vi "SECoP-filterStoredCommand_2.vi"(8 "error in (no error)":errorcluster, 9 "filter action":T1, 10 "filter accessibles":string[](array[string]), 11 "DLL path (in)":T2) -> (0 "error out":errorcluster, 1 "arguments/setvalue":string, 2 "command/parameter path":string, 3 "DLL path (out)":T2, 4 "action":T1, 5 "command id":u64)   [LabVIEW 2023, in "SECoP.lvlib"]
doc: "Call <b>\"SECoP-filterStoredCommand_2.vi\"</b> regulary to check, if there is something to do for selected accessibles only. If yes, it will return successfully with an id, what to do, a parameter/command name and new set value or argument as JSON string.\n\n<b>Note</b>: Keep in mind, that this will filter out only selected accessibles. If there are others, they have to handled with their own filter or use \"SECoP-getStoredCommand_2.vi\".\n\n<b>DLL path</b> input and output of cluster from \"SECoP-Initialize.vi\"\n<b>filter accessibles</b> string list of selected accessibles including node id and module name (format <b>node-id:module:accessible</b>)\n<b>filter action</b> selected action type: <b>any</b> (read/change/do) or special action type\n<b>command id</b> on match: command id for \"SECoP-putCommandAnswer_2.vi\"\n<b>action id</b> on match: action id to handle\n<b>command/parameter path</b> on match: full name of accessible\n<b>arguments/setvalue</b> on match with change or do: JSON input data from SECoP-client"
uses:
  SECoP.lvlib
  SECoP-libraries.ctl
  SECoP-action.ctl
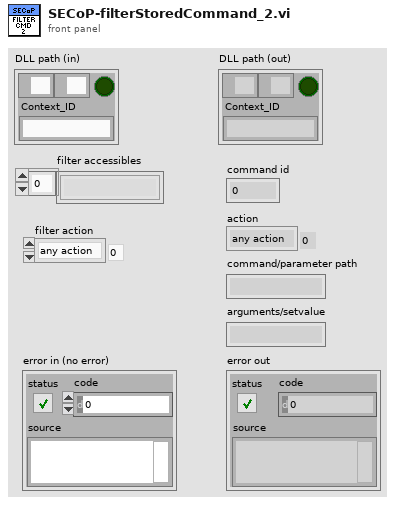
[diagram p1: front panel]
types:
  T1 = typedef "SECoP.lvlib/SECoP-action.ctl" = enum32{"any action", "read", "change", "do cmd"}
  T2 = typedef "SECoP.lvlib/SECoP-libraries.ctl" = cluster{"serverDLL":path, "variantDLL":path, "cleanup_mode":bool, "Context_ID":string}
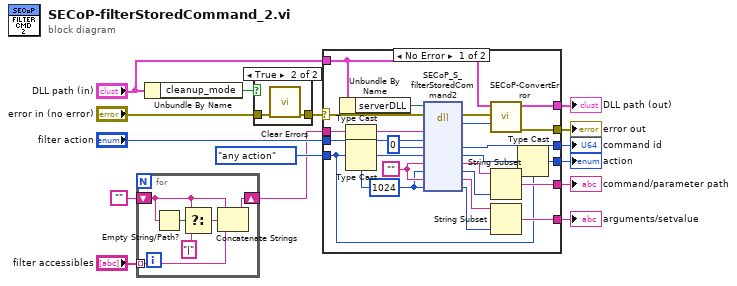
[diagram p0: block diagram]
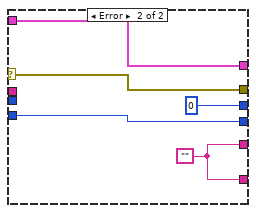
[diagram p3: hidden frame]
diagram:
  n1 = for {
    shift-right: [w16] -> w1
    shift-left: "" -> [w19]
    tunnel: "filter accessibles" -> [w17] mode=indexing
    n2 = Empty String/Path?(string/path=w19) -> (empty?=w21:bool)
    n3 = Select(t=w19, s=w21, f="|") -> (s? t:f=w20:string)
    n4 = Concatenate Strings(w19, w20, w17) -> (w16:string)
  }
  n5 = Unbundle By Name("DLL path (in)") -> ("cleanup_mode"=w10:bool)
  n6 = case shown="True" w10 {
    tunnel: "error in (no error)" -> [w22 w24]
    tunnel: [w22 w23] -> w8
    frame False {
    }
    frame True {
      n7 = call <vilib>:"Clear Errors.vi"("error in (no error)"=w24) -> ("error out"=w23:errorcluster)  [unwired: 5 in, 1 out]
    }
  }
  n8 = case shown="No Error" w8 {
    selector: w8 -> [w46 w52]
    tunnel: "DLL path (in)" -> [w29 w53]
    tunnel: [w47 w53] -> w15
    tunnel: [w48 w52] -> w14
    tunnel: [w37 u64 0 ("id")] -> w13
    tunnel: [w33 w49] -> w7
    tunnel: [w35 w50] -> w12
    tunnel: [w34 w50] -> w11
    tunnel: SECoP-action."any action" ("filter action") -> [w32 w49]
    tunnel: "filter action" -> [w28 _]
    tunnel: w1 -> [w26 _]
    frame No Error {
      w27 = 1024
      w42 = ""
      n9 = Unbundle By Name(w29) -> ("serverDLL"=w30:path)
      n10 = Type Cast(type=w27, x=w28) -> (*(type *) &x=w25:i32)
      n11 = Type Cast(type=w27, x=w32) -> (*(type *) &x=w31:i32)
      n12 = dll-call lib="Z:/Praktische Aufgaben/SECoP-LabVIEW2015/32bit/SECoP32.dll" fn="SECoP_S_filterStoredCommand2"(path in=w30, error in=w46, "szFilterAccessibles"=w26, "iFilterAction"=w25, "pllId"=u64 0 ("id"), "piAction"=w31, "szAccessible"=w42, "piAccessibleSize"=w27, "szValue"=w42, "piValueSize"=w27) -> (error out=w45:errorcluster, "return type"=w44:i32, "pllId"=w37:u64, "piAction"=w36:i32, "szAccessible"=w38:string, "piAccessibleSize"=w39:i32, "szValue"=w41:string, "piValueSize"=w40:i32)  [unwired: 3 in, 1 out]
      n13 = call "SECoP-ConvertError.vi"("return code"=w44, "error in (no error)"=w45, "DLL path (in)"=w29) -> ("error out"=w48:errorcluster, "DLL path (out)"=w47:T2)  [unwired: 7 in]
      n14 = String Subset(string=w38, length (rest)=w39) -> (substring=w35:string)  [unwired: 1 in]
      n15 = String Subset(string=w41, length (rest)=w40) -> (substring=w34:string)  [unwired: 1 in]
      n16 = Type Cast(type=w32, x=w36) -> (*(type *) &x=w33:T1)
    }
    frame Error {
      w50 = ""
    }
  }
  "DLL path (out)" <- w15
  "error out" <- w14
  "command/parameter path" <- w12
  "command id" <- w13
  "arguments/setvalue" <- w11
  "action" <- w7
